vi "Enqueue.vi"(6 "abort? (F)":bool, 7 "last element? (F)":bool, 8 "element":cluster{"cmd":string, "data":variant}, 9 "event priority":T1=enum."normal priority", 10 "is valid? (T)":bool=TRUE, 11 "data in":refnum<class "EventMessengerData.lvclass">) -> (0 "last element?":bool, 3 "data out":refnum<class "EventMessengerData.lvclass">, 4 "aborted?":bool)   [LabVIEW 2019, in "Cmd-Data Event Messenger.lvlib" / "EventMessengerData.lvclass"]
uses:
  EventMessengerData.lvclass
  EventMessengerData.lvclass/EventMessengerData.ctl
  Event Data.ctl
  Cmd-Data Event Messenger.lvlib
  <vilib>/event_ctls.llb/usereventprio.ctl
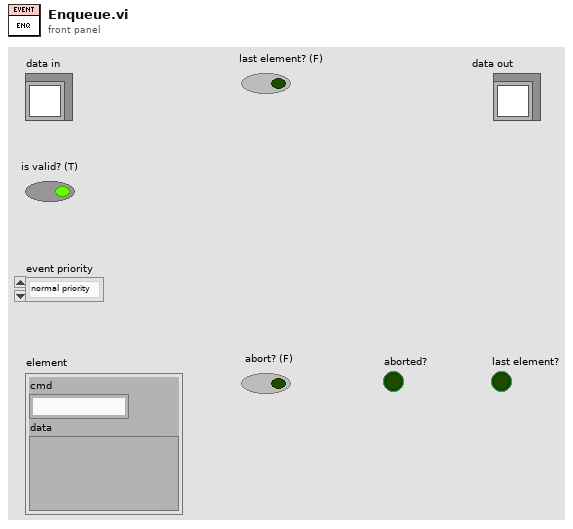
[diagram p1: front panel]
types:
  T1 = typedef "usereventprio.ctl" = enum32{"high priority", "normal priority"}
  T2 = typedef "Cmd-Data Event Messenger.lvlib/Event Data.ctl" = cluster{"msg":cluster{"cmd":string, "data":variant}, "element valid?":bool, "last element?":bool, "aborted?":bool, "priority?":bool}
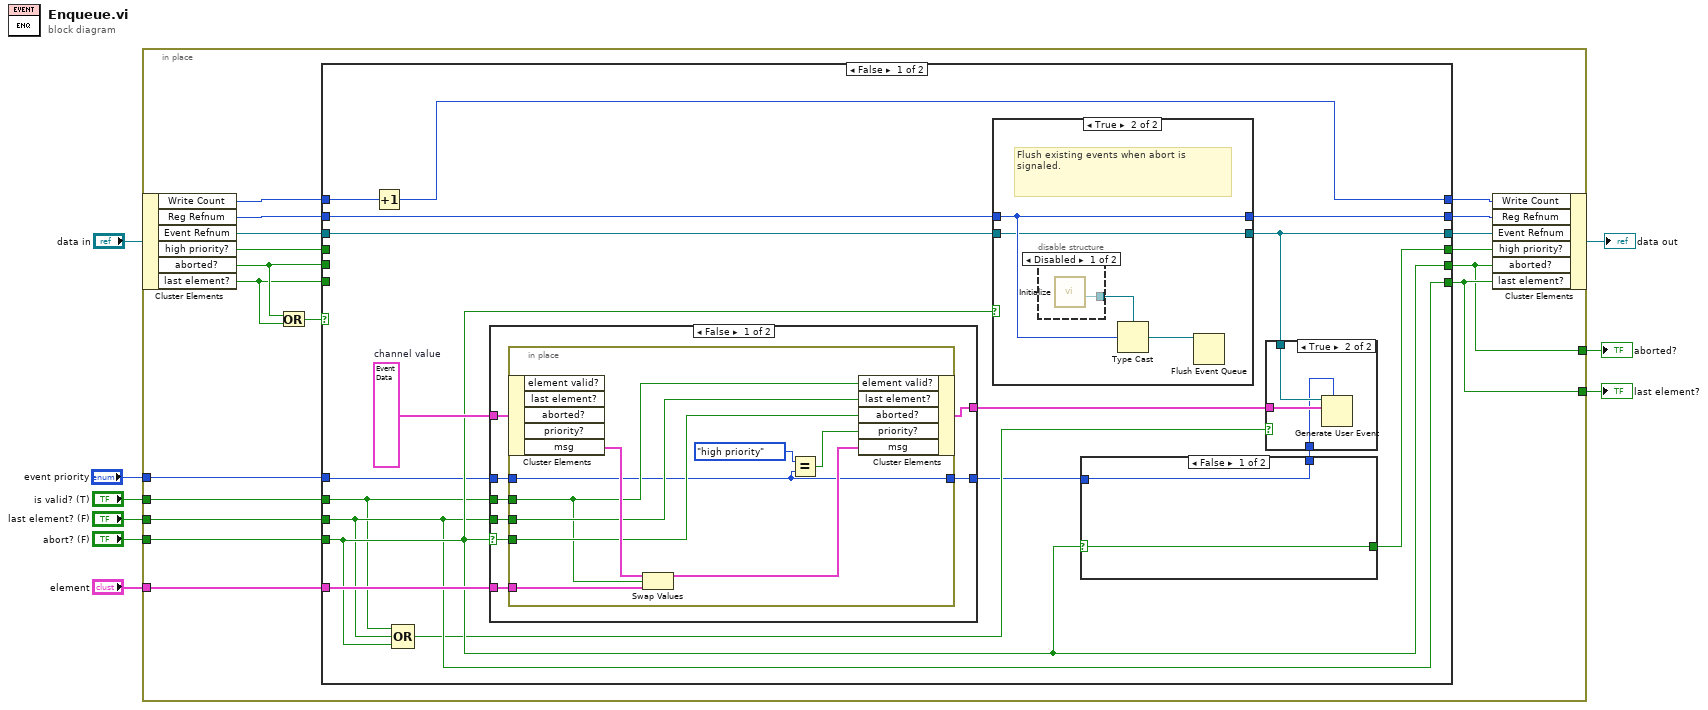
[diagram p0: block diagram]
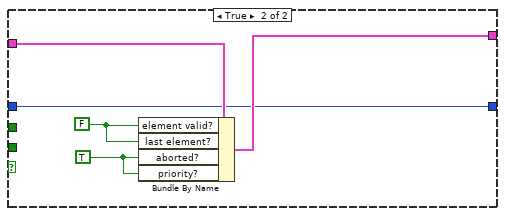
[diagram p2: hidden frame]
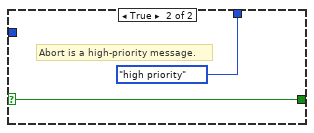
[diagram p4: hidden frame]
diagram:
  n1 = in-place {
    in-place-border: "element" -> [w25]
    in-place-border: "is valid? (T)" -> [w20]
    in-place-border: "last element? (F)" -> [w19]
    in-place-border: "abort? (F)" -> [w18]
    in-place-border: [w14] -> w3
    in-place-border: [w13] -> w2
    in-place-border: "event priority" -> [w10]
    n2 = in-place-cluster #1("data in") -> ("Write Count"=w27:u32, "Reg Refnum"=w21:u32, "Event Refnum"=w24:refnum<user-event>, "high priority?"=w12:bool, "aborted?"=w16:bool, "last element?"=w15:bool)
    n3 = Or(x=w16, y=w15) -> (x .or. y?=w17:bool)
    n4 = case shown="False" w17 {
      tunnel: w27 -> [w44 w86]
      tunnel: [w43 w86] -> w26
      tunnel: w25 -> [w41 _]
      tunnel: w24 -> [w38 w84]
      tunnel: [w39 w84] -> w23
      tunnel: [w37 w85] -> w22
      tunnel: w21 -> [w42 w85]
      tunnel: [w34 w83] -> w13
      tunnel: w20 -> [w32 _]
      tunnel: w19 -> [w33 _]
      tunnel: w18 -> [w34 _]
      tunnel: w16 -> [_ w83]
      tunnel: [w33 w82] -> w14
      tunnel: w15 -> [_ w82]
      tunnel: w10 -> [w29 _]
      tunnel: w12 -> [_ w81]
      tunnel: [w30 w81] -> w11
      frame False {
        w36 = T2 {"msg"={"cmd"="", "data"=variant}, "element valid?"=FALSE, "last element?"=FALSE, "aborted?"=FALSE, "priority?"=FALSE}  # channel value
        n5 = Increment(x=w44) -> (x+1=w43:u32)
        n6 = Compound Arithmetic op=OR(w32, w33, w34) -> (w31:bool)
        n7 = case shown="False" w34 {
          selector: w34 -> [w48 _]
          tunnel: w32 -> [w52 _]
          tunnel: w41 -> [w51 _]
          tunnel: [w50 w65] -> w40
          tunnel: w36 -> [w49 w66]
          tunnel: w33 -> [w47 _]
          tunnel: w29 -> [w46 w63]
          tunnel: [w45 w63] -> w28
          frame False {
            n8 = in-place {
              in-place-border: w52 -> [w56]
              in-place-border: w47 -> [w57]
              in-place-border: w48 -> [w58]
              in-place-border: w51 -> [w60]
              in-place-border: w46 -> [w53]
              in-place-border: [w53] -> w45
              n9 = in-place-cluster #2(w49) -> ("msg"=w61:cluster{"cmd":string, "data":variant})  [unwired: 4 out]
              n10 = Swap Values(12:w61, 13:w56, 14:w60) -> (1:w59:cluster{"cmd":string, "data":variant})  [unwired: 1 out]
              n11 = Equal?(x=usereventprio."high priority" ("y"), y=w53) -> (x = y?=w54:bool)
              n12 = in-place-cluster #2("element valid?"=w56, "last element?"=w57, "aborted?"=w58, "priority?"=w54, "msg"=w59) -> (w50:T2)
            }
          }
          frame True {
            w62 = TRUE ("last element?")
            w64 = FALSE ("element valid?")
            n13 = Bundle By Name(cluster=w66, "element valid?"=w64, "last element?"=w64, "aborted?"=w62, "priority?"=w62) -> (w65:T2)
          }
        }
        n14 = case shown="True" w34 {
          tunnel: [w75 w77] -> w39
          tunnel: w38 -> [w75 w77]
          tunnel: [w74 w79] -> w37
          tunnel: w42 -> [w74 w79]
          frame False {
            # "If not aborting, keep using the same refnum as previous Write calls."
          }
          frame True {
            # "Flush existing events when abort is signaled."
            n15 = disable-structure shown="Disabled" {
              disable-tunnel: [w80 _] -> w76
              frame Disabled {
                n16 = call "Initialize.vi"() -> ("Event Registration Refnum"=w80:refnum<event-registration>)  [unwired: 10 in, 1 out]
              }
              frame Enabled {
              }
            }
            n17 = Type Cast(type=w76, x=w79) -> (*(type *) &x=w78:refnum<event-registration>)
            n18 = Flush Event Queue(0:w78) -> ()  [unwired: 5 in, 3 out]
          }
        }
        n19 = case shown="False" w34 {
          selector: w34 -> [w70 w72]
          tunnel: w28 -> [w71 _]
          tunnel: [w71 usereventprio."high priority" ("event priority")] -> w35
          tunnel: [w70 w72] -> w30
          frame False {
          }
          frame True {
            # "Abort is a high-priority message."
          }
        }
        n20 = case shown="True" w31 {
          tunnel: w40 -> [_ w69]
          tunnel: w39 -> [_ w68]
          tunnel: w35 -> [_ w67]
          frame False {
          }
          frame True {
            n21 = Generate User Event(priority (normal)=w67, user event=w68, event data cluster=w69) -> ()  [unwired: 1 in, 2 out]
          }
        }
      }
      frame True {
        # "If aborted or last element has already been sent on previous writes then this channel is done until it gets re-initialized, so don't do anything now."
      }
    }
    n22 = in-place-cluster #1("Write Count"=w26, "Reg Refnum"=w22, "Event Refnum"=w23, "high priority?"=w11, "aborted?"=w13, "last element?"=w14) -> (→"data out":refnum<class "EventMessengerData.lvclass">)
  }
  "aborted?" <- w2
  "last element?" <- w3
